vi "LJT4_V2T.vi"(8 "CJC (K)":dbl, 11 "voltage_array":dbl[](array[numeric])) -> (0 "array_mV":dbl[](array[numeric]), 1 "array_T_F":dbl[](array[numeric]), 2 "array_T_C":dbl[](array[numeric]), 3 "array_T_K":dbl[](array[numeric]))   [LabVIEW 2019]
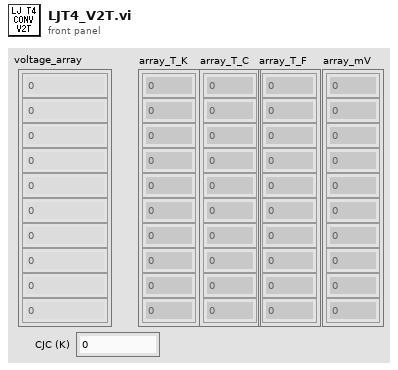
[diagram p1: front panel]
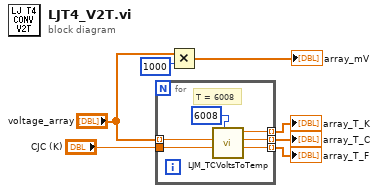
[diagram p0: block diagram]
diagram:
  n1 = for {
    tunnel: "voltage_array" -> [w9] mode=indexing
    tunnel: [w10] -> w7 mode=indexing
    tunnel: [w12] -> w5 mode=indexing
    tunnel: [w11] -> w6 mode=indexing
    tunnel: "CJC (K)" -> [w8]
    # "T = 6008"
    n2 = call "LJM_TCVoltsToTemp.vi"("TCType"=6008, "CJTempK"=w8, "TCVolts"=w9) -> ("TCTempF"=w10:dbl, "TCTempC"=w11:dbl, "TCTempK"=w12:dbl)  [unwired: 5 in, 1 out]
  }
  "array_T_F" <- w7
  "array_T_C" <- w6
  "array_T_K" <- w5
  n3 = Multiply(x="voltage_array", y=1000) -> (x*y=→"array_mV":dbl[])
